vi "Set delay position to zero.vi"(8 "error in (no error)":errorcluster, 10 "Set Delay Position to Zero":bool, 11 "Delay Line":enum16{"K1", "K2", "K3"}(ring)) -> (0 "error out":errorcluster)   [LabVIEW 2009]
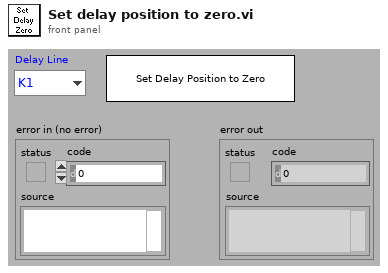
[diagram p1: front panel]
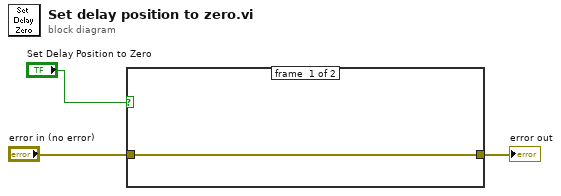
[diagram p0: block diagram]
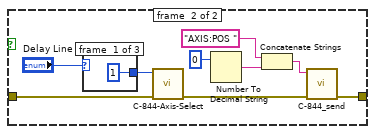
[diagram p2: hidden frame]
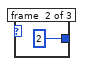
[diagram p3: hidden frame]
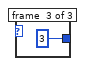
[diagram p4: hidden frame]
diagram:
  n1 = case shown="True" "Set Delay Position to Zero" {
    tunnel: [w4 w6] -> w3
    tunnel: "error in (no error)" -> [w4 w5]
    frame #0 {
    }
    frame #1 {
      n2 = case shown="\"K1\"" "Delay Line" {
        tunnel: [u8 1 u8 2 u8 3] -> w7
        frame #0 {
        }
        frame #1 {
        }
        frame #2 {
        }
      }
      n3 = call "C-844-Axis-Select.vi"("error in (no error)"=w5, "Axis Select"=w7) -> ("error out"=w13:errorcluster)  [unwired: 8 in, 1 out]
      n4 = Number To Decimal String(number=0) -> (decimal integer string=w12:string)  [unwired: 1 in]
      n5 = Concatenate Strings("AXIS:POS ", w12) -> (w11:string)
      n6 = call "C-844_send.vi"("error in (no error)"=w13, "Command"=w11) -> ("error out"=w6:errorcluster)  [unwired: 7 in, 2 out]
    }
  }
  "error out" <- w3
